vi "Read User Timestamps From Disk.vi"(0 "file path":path, 11 "error in (no error)":errorcluster) -> (4 "user timestamps":T1[](array[typedef]), 15 "error out":errorcluster)   [LabVIEW 2023, in "GettingStarted_Common_148X_Host.lvlib"]
uses:
  GettingStarted_Common_148X_Host.lvlib
  <instrlib>/FlexRIO/CSI-2/v2/FPGA/Types/User Timestamp.ctl
  <instrlib>/FlexRIO/CSI-2/v2/FPGA/Types/Timestamp ID.ctl
  <instrlib>/FlexRIO/CSI-2/v2/FPGA/Types/Raw Timestamp.ctl
  <instrlib>/FlexRIO/CSI-2/v2/Host/subVIs/Convert Raw Timestamp to User Timestamp.vi
  <instrlib>/FlexRIO/CSI-2/v2/FPGA/NI CSI-2 API FPGA v2.lvlib
  <instrlib>/FlexRIO/CSI-2/v2/Host/NI CSI-2 API Host v2.lvlib
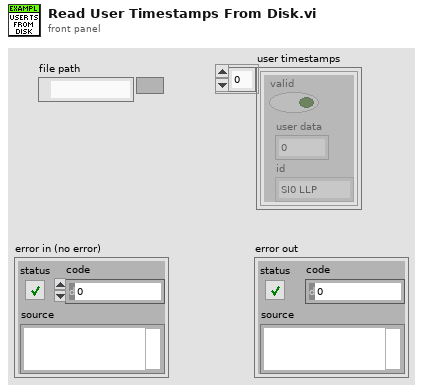
[diagram p1: front panel]
types:
  T1 = typedef "NI CSI-2 API FPGA v2.lvlib/User Timestamp.ctl" = cluster{"valid":bool, "user data":fxp<+,58,58>, "id":T2}
  T2 = typedef "NI CSI-2 API FPGA v2.lvlib/Timestamp ID.ctl" = enum8{"SI0 LLP", "SI1 LLP", "SI2 LLP", "SI3 LLP", "SI4 LLP", "SI5 LLP", "SI6 LLP", "SI7 LLP", "SO0 LLP", "SO1 LLP", "SO2 LLP", "SO3 LLP", "SO4 LLP", "SO5 LLP", "SO6 LLP", "SO7 LLP", "Ser0 GPIO Bank", "Ser1 GPIO Bank", "Ser2 GPIO Bank", "Ser3 GPIO Bank", "Ser4 GPIO Bank", "Ser5 GPIO Bank", "Ser6 GPIO Bank", "Ser7 GPIO Bank", "Des0 GPIO Bank", "Des1 GPIO Bank", "Des2 GPIO Bank", "Des3 GPIO Bank", "Des4 GPIO Bank", "Des5 GPIO Bank", "Des6 GPIO Bank", "Des7 GPIO Bank", "User0", "User1", "User2", "User3", "User4", "User5", "User6", "User7", "User8", "User9", "User10", "User11", "User12", "User13", "User14", "User15", "User16", "User17", "User18", "User19", "User20", "User21", "User22", "User23", "User24", "User25", "User26", "User27", "User28", "User29", "User30", "User31"}
  T3 = enum16{"open", "open or create", "create or replace", "create", "open (read-only)"}
  T4 = typedef "NI CSI-2 API FPGA v2.lvlib/Raw Timestamp.ctl" = cluster{"timestamp":u64, "valid":bool}
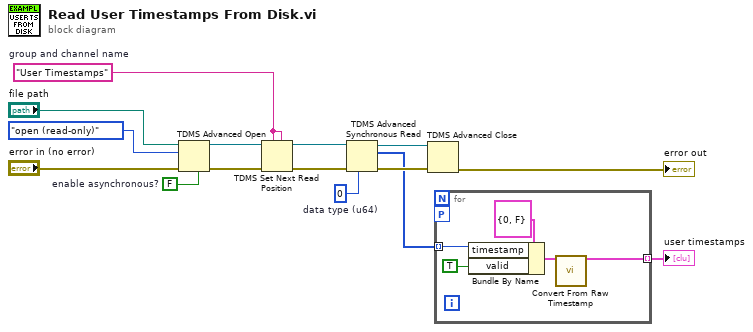
[diagram p0: block diagram]
diagram:
  w2 = "User Timestamps"  # group and channel name
  w7 = FALSE  # enable asynchronous?
  w13 = u64 0  # data type (u64)
  n1 = TDMS Advanced Open(4:w7, 8:"error in (no error)", 10:T3."open (read-only)" ("operation (0:open)"), 11:"file path") -> (0:w6:errorcluster, 3:w3:refnum<k34>)  [unwired: 1 in, 1 out]
  n2 = TDMS Set Next Read Position(5:w2, 7:w2, 8:w6, 11:w3) -> (0:w5:errorcluster, 3:w4:refnum<k34>)  [unwired: 2 in]
  n3 = TDMS Advanced Synchronous Read(6:w13, 8:w5, 11:w4) -> (0:w14:errorcluster, 2:w8:u64[], 3:w15:refnum<k34>)  [unwired: 1 in, 1 out]
  n4 = TDMS Advanced Close(8:w14, 11:w15) -> (0:→"error out":errorcluster)  [unwired: 2 in, 1 out]
  n5 = for {
    tunnel: w8 -> [w18] mode=indexing
    tunnel: [w17] -> w1 mode=indexing
    workers-P: _ -> [_]
    n6 = Bundle By Name(cluster=T4 {"timestamp"=0, "valid"=FALSE} ("raw timestamp"), "timestamp"=w18, "valid"=TRUE) -> (w19:T4)
    n7 = call-poly <instrlib>:"Convert From Raw Timestamp.vi"("raw timestamp"=w19) -> ("user timestamp"=w17:T1)  [unwired: 14 in]
  }
  "user timestamps" <- w1
